vi "Helper - String to Log String.vi"(9 "Input":string, 10 "Selector":string, 11 "PrevString":string) -> (3 "Output":string)   [LabVIEW 2011]
doc: "Part of Helper - Data to String.vi. Look there for more details."
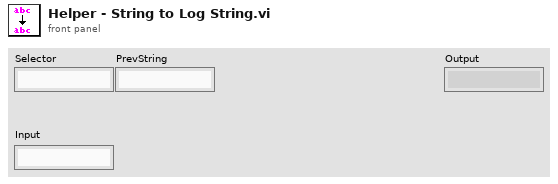
[diagram p1: front panel]
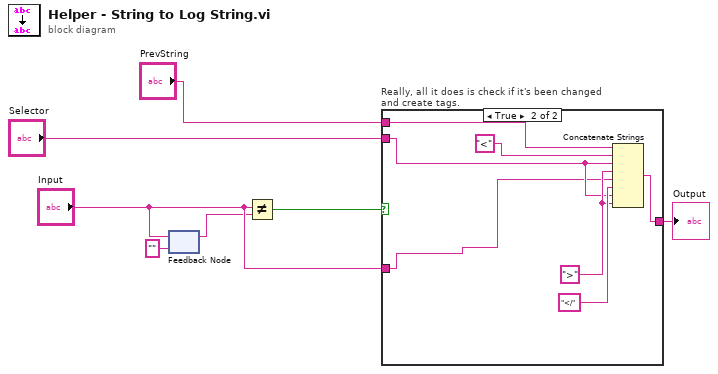
[diagram p0: block diagram]
diagram:
  n1 = feedback-in #1("Input") -> ()
  n2 = feedback #1("" ("Input")) -> (w2:string)
  n3 = Not Equal?(x="Input", y=w2) -> (x != y?=w4:bool)
  n4 = case "Really, all it does is check if it's been changed and create tags." shown="True" w4 {
    tunnel: [w8 w15] -> w6
    tunnel: "Selector" -> [_ w10]
    tunnel: "Input" -> [_ w9]
    tunnel: "PrevString" -> [w8 w11]
    frame False {
    }
    frame True {
      w12 = ">" ("string")
      n5 = Concatenate Strings(w11, "<" ("string"), w10, w12, w9, "</" ("string"), w10, w12) -> (w15:string)
    }
  }
  "Output" <- w6
